vi "Send File to Server.vi"(8 "error in (no error)":errorcluster, 10 "file to send":path, 11 "Logger in":refnum<class "Logger.lvclass">) -> (0 "error out":errorcluster, 3 "Logger out":refnum<class "Logger.lvclass">)   [LabVIEW 2017, in "Logger.lvlib" / "Logger.lvclass"]
uses:
  Logger.lvclass
  Logger.lvclass/Logger.ctl
  <vilib>/Skyline/File/File/Send File.vi
  <vilib>/Skyline/File/File/NI Skyline File.lvclass
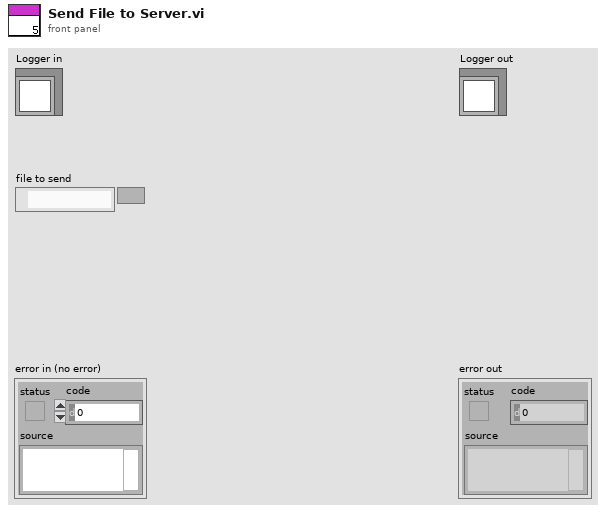
[diagram p1: front panel]
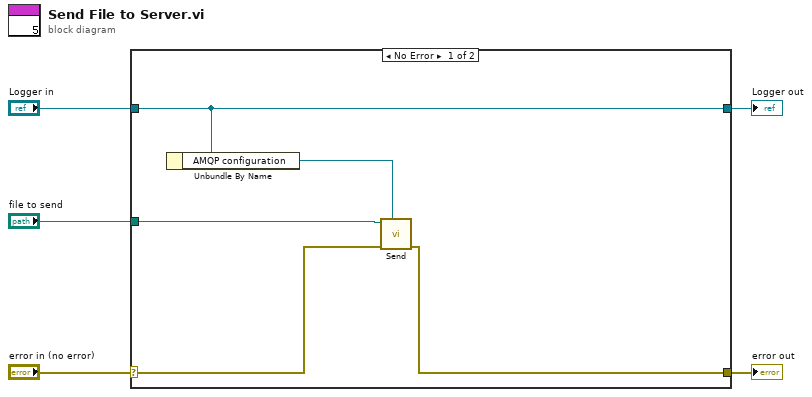
[diagram p0: block diagram]
diagram:
  n1 = case shown="No Error" "error in (no error)" {
    selector: "error in (no error)" -> [w7 w12]
    tunnel: [w6 w12] -> w4
    tunnel: [w9 w11] -> w2
    tunnel: "Logger in" -> [w9 w11]
    tunnel: "file to send" -> [w10 _]
    frame No Error {
      n2 = Unbundle By Name(w9) -> ("AMQP configuration"=w8:refnum<class "NI Skyline Configuration AMQP.lvclass">)
      n3 = call-poly <vilib>:"Send.vi"("AMQP configuration"=w8, "error in (no error)"=w7, "path"=w10) -> ("error out"=w6:errorcluster)  [unwired: 6 in, 1 out]
    }
    frame Error {
    }
  }
  "error out" <- w4
  "Logger out" <- w2
